vi "FourierTransform.vi"(2 "Cutoff (s)":dbl=-1.0, 3 "Time Data":dbl[](array[numeric]), 4 "time per sample":dbl) -> (0 "Spectrum":cluster{dbl, "df":dbl, dbl[]}(graph), 1 "FFT":cluster{dbl, "df":dbl, "FFT {X}":cdb[]})   [LabVIEW 2014]
uses:
  <vilib>/Analysis/2dsp.llb/Real FFT.vi
  <vilib>/Analysis/NI_AALPro.lvlib
  <vilib>/Analysis/NI_AALBase.lvlib
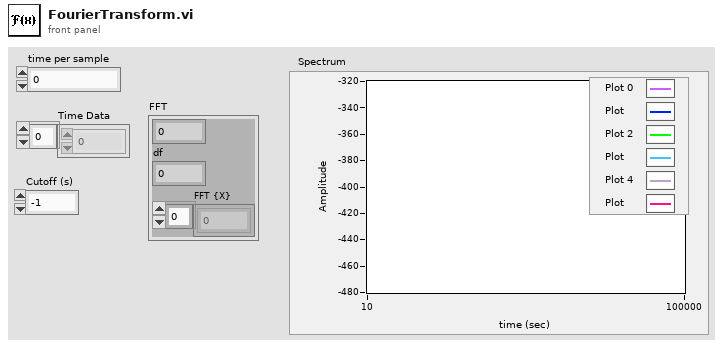
[diagram p1: front panel]
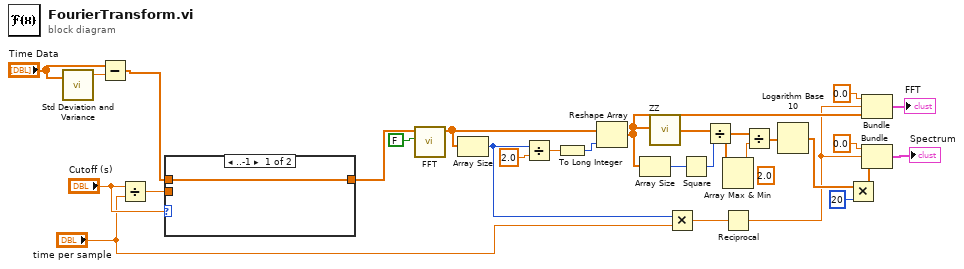
[diagram p0: block diagram]
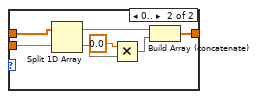
[diagram p2: hidden frame]
diagram:
  (unwired) 2.0
  n1 = call <vilib>:"Std Deviation and Variance.vi"("X"="Time Data") -> ("mean"=w16:dbl)  [unwired: 1 in, 2 out]
  n2 = Subtract(x="Time Data", y=w16) -> (x-y=w12:dbl[])
  n3 = Divide(x="Cutoff (s)", y="time per sample") -> (x/y=w20:dbl)
  n4 = case shown="..-1" "Cutoff (s)" {
    tunnel: [w30 w31] -> w19
    tunnel: w12 -> [w30 w34]
    tunnel: w20 -> [_ w33]
    frame ..-1 {
    }
    frame 0.. {
      n5 = Split 1D Array(array=w34, index=w33) -> (first subarray=w32:dbl[], second subarray=w35:dbl[])
      n6 = Multiply(x=0.0, y=w35) -> (x*y=w36:dbl[])
      n7 = Build Array (concatenate)(w32, w36) -> (w31:dbl[])
    }
  }
  n8 = call-poly <vilib>:"FFT.vi"("shift?"=FALSE, "X"=w19) -> ("FFT {X}"=w24:cdb[])  [unwired: 8 in, 1 out]
  n9 = Array Size(array=w24) -> (size(s)=w5:i32)
  n10 = Divide(x=w5, y=2.0) -> (x/y=w22:dbl)
  n11 = To Long Integer(number=w22) -> (32bit integer=w23:i32)
  n12 = Reshape Array(w24, w23) -> (w10:cdb[])
  n13 = Array Size(array=w10) -> (size(s)=w27:i32)
  n14 = call <userlib>:"ZZ.vi"("P"=w10) -> ("PP*"=w11:dbl[])
  n15 = Multiply(x=w5, y="time per sample") -> (x*y=w6:dbl)
  n16 = Square(x=w27) -> (x^2=w26:i32)
  n17 = Divide(x=w11, y=w26) -> (x/y=w2:dbl[])
  n18 = Array Max & Min(array=w2) -> (max value=w1:dbl)  [unwired: 3 out]
  n19 = Reciprocal(x=w6) -> (1/x=w3:dbl)
  n20 = Divide(x=w2, y=w1) -> (x/y=w8:dbl[])
  n21 = Logarithm Base 10(1:w8) -> (0:w14:dbl[])
  n22 = Multiply(x=w14, y=20) -> (x*y=w9:dbl[])
  n23 = Bundle(0.0, w3, "FFT {X}"=w10) -> (→"FFT":cluster{dbl, dbl, "FFT {X}":cdb[]})  [unwired: 1 in]
  n24 = Bundle(0.0, w3, w9) -> (→"Spectrum":cluster{dbl, dbl, dbl[]})  [unwired: 1 in]
